vi "Set GE 5565PIORC.vi"(10 "GE 5565PIORC":refnum<class "GE 5565PIORC.lvclass">, 11 "GE Reflective Memory in":refnum<class "GE Reflective Memory Transceiver.lvclass">) -> (3 "GE Reflective Memory out":refnum<class "GE Reflective Memory Transceiver.lvclass">)   [LabVIEW 2017, in "GE Reflective Memory.lvlib" / "GE Reflective Memory Transceiver.lvclass"]
uses:
  GE Reflective Memory Transceiver.lvclass
  <vilib>/NI/GE Reflective Memory Driver/GE 5565PIORC.lvclass
  GE Reflective Memory Transceiver.lvclass/GE Reflective Memory Transceiver.ctl
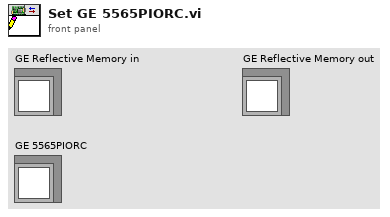
[diagram p1: front panel]
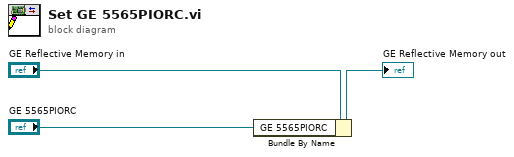
[diagram p0: block diagram]
diagram:
  n1 = Bundle By Name(cluster="GE Reflective Memory in", "GE 5565PIORC"="GE 5565PIORC") -> (→"GE Reflective Memory out":refnum<class "GE Reflective Memory Transceiver.lvclass">)
